vi "Discover Inst Model.vi"(8 "error in":errorcluster {"code" format="%.0x"}, 11 "Session In":refnum<visa-resource-name>="GPIB0::11::INSTR") -> (0 "error out":errorcluster {"code" format="%.0x"}, 2 "Model #":string, 3 "Session Out":refnum<visa-resource-name>)   [LabVIEW 2018]
doc: "Launches the Instrument I/O Assistant, which you can use to communicate with message-based instruments and graphically parse the response. For example you can communicate with an instrument that uses a serial, Ethernet, or GPIB interface."
panel:
  out "token4":string
  out "token3":string
  out "token":string
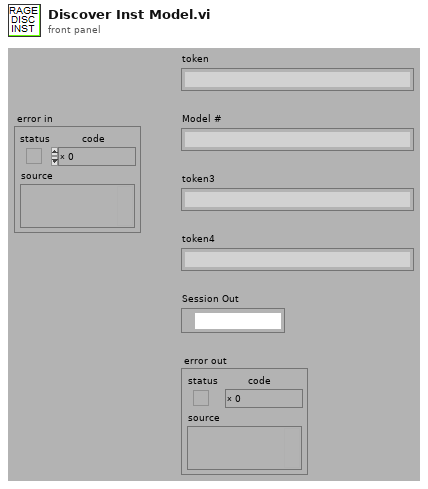
[diagram p1: front panel]
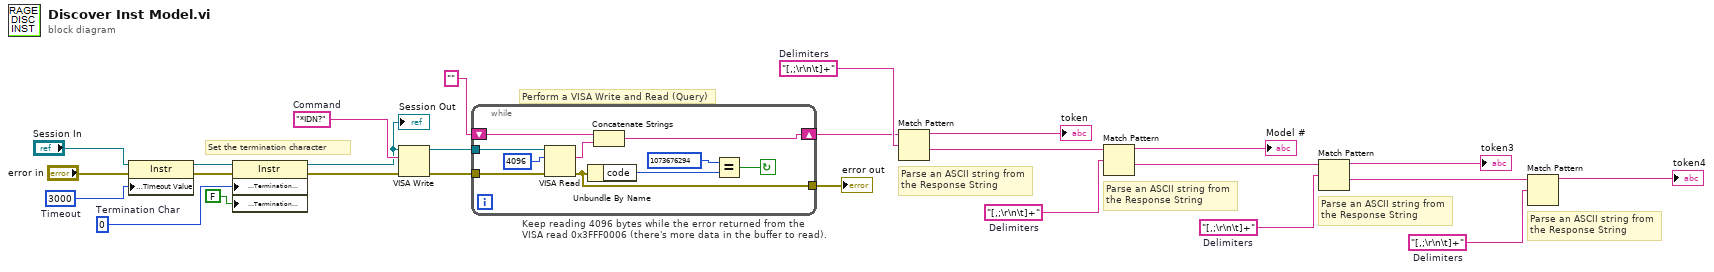
[diagram p0: block diagram]
diagram:
  w3 = "[,;\r\n\t]+"  # Delimiters
  w6 = "[,;\r\n\t]+"  # Delimiters
  w9 = "[,;\r\n\t]+"  # Delimiters
  w12 = "[,;\r\n\t]+"  # Delimiters
  w14 = "*IDN?"  # Command
  w21 = u8 0  # Termination Char
  w26 = u32 3000  # Timeout
  # "Parse an ASCII string from the Response String"
  # "Parse an ASCII string from the Response String"
  # "Parse an ASCII string from the Response String"
  # "Parse an ASCII string from the Response String"
  # "Perform a VISA Write and Read (Query)"
  # "Keep reading 4096 bytes while the error returned from the\nVISA read 0x3FFF0006 (there's more data in the buffer to read)."
  # "Set the termination character"
  n1 = property class="Instr"(reference="Session In", error in="error in", "General Settings:Timeout Value"=w26) -> (reference out=w20:refnum<visa-resource-name>, error out=w23:errorcluster)
  n2 = property class="Instr"(reference=w20, error in=w23, "Message Based Settings:Termination Character"=w21, "Message Based Settings:Termination Character Enable"=FALSE ("enable")) -> (reference out=w1:refnum<visa-resource-name>, error out=w22:errorcluster)
  "Session Out" <- w1
  n3 = VISA Write(VISA resource name=w1, write buffer=w14, error in (no error)=w22) -> (VISA resource name out=w18:refnum<visa-resource-name>, error out=w17:errorcluster)  [unwired: 1 out]
  n4 = while {
    tunnel: w18 -> [w33]
    shift-right: [w27] -> w11
    shift-left: "" -> [w32]
    tunnel: w17 -> [w30]
    tunnel: [w29] -> w16
    stop <- w28 continue-if-true
    n5 = VISA Read(VISA resource name=w33, byte count=u32 4096 ("byte count (0)"), error in (no error)=w30) -> (read buffer=w31:string, error out=w29:errorcluster)  [unwired: 2 out]
    n6 = Unbundle By Name(w29) -> ("code"=w35:i32)
    n7 = Concatenate Strings(w32, w31) -> (w27:string)
    n8 = Equal?(x=1073676294, y=w35) -> (x = y?=w28:bool)
  }
  "error out" <- w16
  n9 = Match Pattern(string=w11, regular expression=w12) -> (before substring=→"token":string, after substring=w8:string)  [unwired: 3 out]
  n10 = Match Pattern(string=w8, regular expression=w9) -> (before substring=→"Model #":string, after substring=w5:string)  [unwired: 3 out]
  n11 = Match Pattern(string=w5, regular expression=w6) -> (before substring=→"token3":string, after substring=w2:string)  [unwired: 3 out]
  n12 = Match Pattern(string=w2, regular expression=w3) -> (before substring=→"token4":string)  [unwired: 4 out]
